vi "CHS_TRAJECTORY_GET_REL_TRAJ.vi"() -> (3 "Relative_Trajectory":T1)   [LabVIEW 2019]
uses:
  <vilib>/Rock Robotics/WPI/ThirdParty/ChoreoLib/TypeDef/ChoreoTrajectory.ctl
  <vilib>/Rock Robotics/WPI/ThirdParty/ChoreoLib/TypeDef/ChoreoTrajectoryState.ctl
  CHS_TRAJECTORY_GLOBALS.vi
  <vilib>/Rock Robotics/WPI/ThirdParty/ChoreoLib/ChoreoLib.lvlib
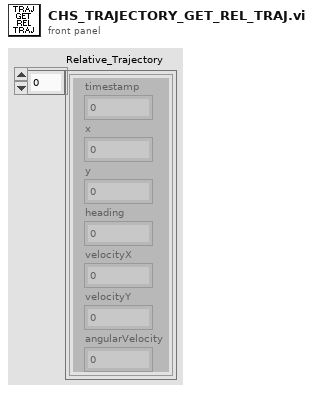
[diagram p1: front panel]
types:
  T1 = typedef "ChoreoLib.lvlib/ChoreoTrajectory.ctl" = T2[]
  T2 = typedef "ChoreoLib.lvlib/ChoreoTrajectoryState.ctl" = cluster{"timestamp":dbl, "x":dbl, "y":dbl, "heading":dbl, "velocityX":dbl, "velocityY":dbl, "angularVelocity":dbl}
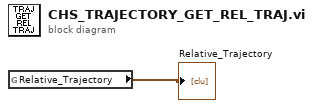
[diagram p0: block diagram]
diagram:
  n1 = global read "CHS_TRAJECTORY_GLOBALS.vi" "Relative_Trajectory"() -> (→"Relative_Trajectory":T1)
